vi "RSZVB Get Virtual Transform Port Pair State.vi"(7 "Port Pair (1)":i32=1, 8 "error in (no error)":errorcluster {"code" format="%.0x"}, 9 "Function Type (Deembedding)":i32(ring) items=["Deembedding", "Embedding"], 10 "Channel (1)":i32=1, 11 "VISA session":refnum<visa-resource-name>) -> (0 "error out":errorcluster {"code" format="%.0x"}, 2 "State":bool, 3 "dup VISA session":refnum<visa-resource-name>)   [LabVIEW 2011]
doc: "This VI queries the state of the deembedding/embedding function for for port pairs.\n\nRemote-control command(s):\nCALCulate<Ch>:TRANsform:VNETworks:PPAir:DEEMbedding<List_idx>[:STATe]?\nCALCulate<Ch>:TRANsform:VNETworks:PPAir:EMBedding<List_idx>[:STATe]?"
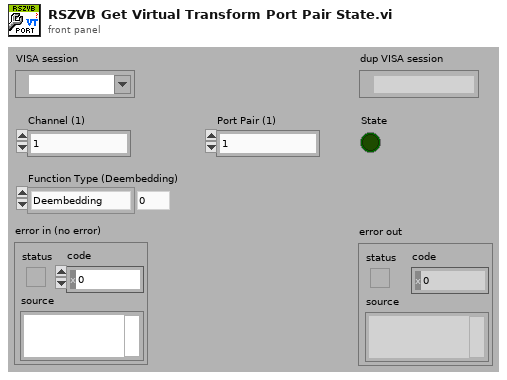
[diagram p1: front panel]
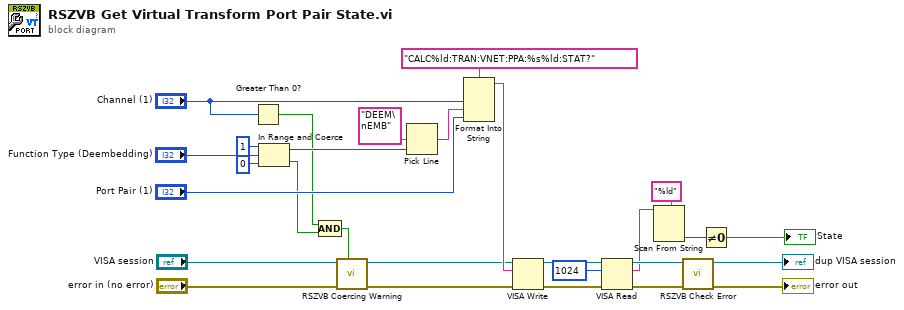
[diagram p0: block diagram]
diagram:
  n1 = Greater Than 0?(x="Channel (1)") -> (x > 0?=w5:bool)
  n2 = In Range and Coerce(upper limit=1, x="Function Type (Deembedding)", lower limit=0) -> (coerced(x)=w8:i32, In Range?=w4:bool)
  n3 = Compound Arithmetic op=AND(w5, w4) -> (w3:bool)
  n4 = call "RSZVB Coercing Warning.vi"("In Range?"=w3, "error in (no error)"="error in (no error)", "VISA session"="VISA session") -> ("error out"=w27:errorcluster, "dup VISA session"=w26:refnum<visa-resource-name>)  [unwired: 7 in]
  n5 = Pick Line(multi-line string="DEEM\nEMB", line index=w8) -> (output string=w7:string)  [unwired: 1 in]
  n6 = Format Into String(format string="CALC%ld:TRAN:VNET:PPA:%s%ld:STAT?", "Channel (1)", w7, "Port Pair (1)") -> (resulting string=w28:string)  [unwired: 2 in, 1 out]
  n7 = VISA Write(VISA resource name=w26, write buffer=w28, error in (no error)=w27) -> (VISA resource name out=w21:refnum<visa-resource-name>, error out=w20:errorcluster)  [unwired: 1 out]
  n8 = VISA Read(VISA resource name=w21, byte count=u32 1024 ("byte count (0)"), error in (no error)=w20) -> (VISA resource name out=w23:refnum<visa-resource-name>, read buffer=w17:string, error out=w24:errorcluster)  [unwired: 1 out]
  n9 = Scan From String(format string="%ld", input string=w17) -> (output 1=w18:i32)  [unwired: 3 in, 3 out]
  n10 = call "RSZVB Check Error.vi"("error in (no error)"=w24, "VISA session"=w23) -> ("error out"=→"error out":errorcluster, "dup VISA session"=→"dup VISA session":refnum<visa-resource-name>)  [unwired: 8 in]
  n11 = Not Equal To 0?(x=w18) -> (x != 0?=→"State":bool)
